vi "Car Wash.vi"() -> ()   [LabVIEW 2024]
doc: "Car wash\n\nWash entry : indicate empty or in use\nUser selects car wash options \nStart option\nCar wash indicator shows current step in car wash\nshows the elapsed time on indicator\nVehicle out of position indicator -> elapsed timer pause\n\nProgram start\nAll controls enabled\nWash entry green\n-> Wash vacant\nAll wash indicators turned off; elapsed time =0\nCar position slider Entry\n\nSelects wash options\nHigh pressure is the default\nStart -> starts the selected car wash options one by one\n\nShould disable all the wash options after start\nWash entry LED red -> Wash in Progress\n\nCheck if the car is in position\n\nUpon completing car wash step; if car is in position, go to next car wash step\n\nOnce all car wash steps are complete, vehicle out of position should turn green. User moves car position slider to exit car wash indicators off\nCar position slider -> Entry\nWash entry green and wash vacant\nWash entry cinsole options enabled"
uses:
  Controls/Wash Options.ctl
  Controls/Car Wash Indicators.ctl
  Controls/States.ctl
panel:
  out "Output":T2 {"Elapsed Time" format="%0.2f"}
  in  "Start":bool
  in  "stop":bool
  in  "Wash Options":T3
  in  "Car Position Slider":u8(slide) max=3 scale=0.0..4.0
  # "Entry Console"
  # "Car Wash Display"
  # "Car Position Simulation"
  # "Pre-Soak\nH-P Wash\nL-P Wax\nSpot Free Rinse"
  # "Underbody Wash\nBug Remover"
  # "Tire Shine\nAir Dry"
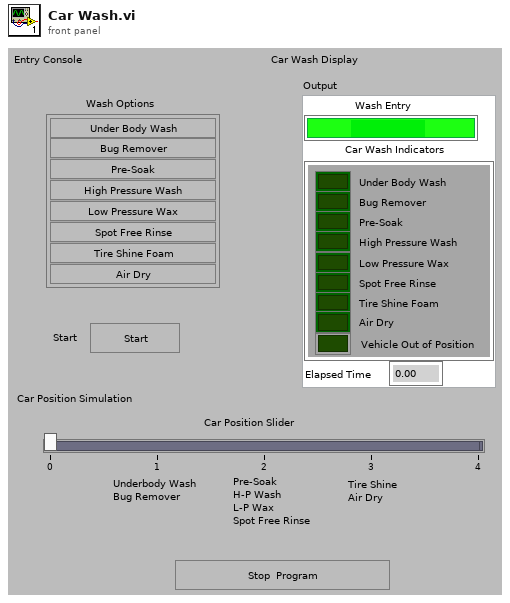
[diagram p1: front panel]
types:
  T1 = typedef "Car Wash Indicators.ctl" = cluster{"Under Body Wash":bool, "Bug Remover":bool, "Pre-Soak":bool, "High Pressure Wash":bool, "Low Pressure Wax":bool, "Spot Free Rinse":bool, "Tire Shine Foam":bool, "Air Dry":bool, "Vehicle Out of Position":bool}
  T2 = cluster{"Wash Entry":bool, "Car Wash Indicators":T1, "Elapsed Time":dbl}
  T3 = typedef "Wash Options.ctl" = cluster{"Underbody Wash":bool, "Bug Remover":bool, "Pre-Soak":bool, "High Pressure Wash":bool, "Low Pressure Wax":bool, "Spot Free Rinse":bool, "Tire Shine Foam":bool, "Air Dry":bool}
  T4 = cluster{"Start":refnum<vi>, "Wash Options":refnum<vi>, "Car Position Slider":refnum<vi>, "Wash Entry":refnum<vi>, "Elapsed Time":refnum<vi>}
  T5 = typedef "States.ctl" = enum16{"Initialize", "Wait for Event", "Under Body Wash", "Bug Remover", "Pre-Soak", "High Pressure Wash", "Low Pressure Wax", "Spot Free Rinse", "Tire Shine Foam", "Exit", "Air Dry", "Stop"}
  T6 = enum8{"Enabled", "Disabled", "Disabled and Grayed Out"}
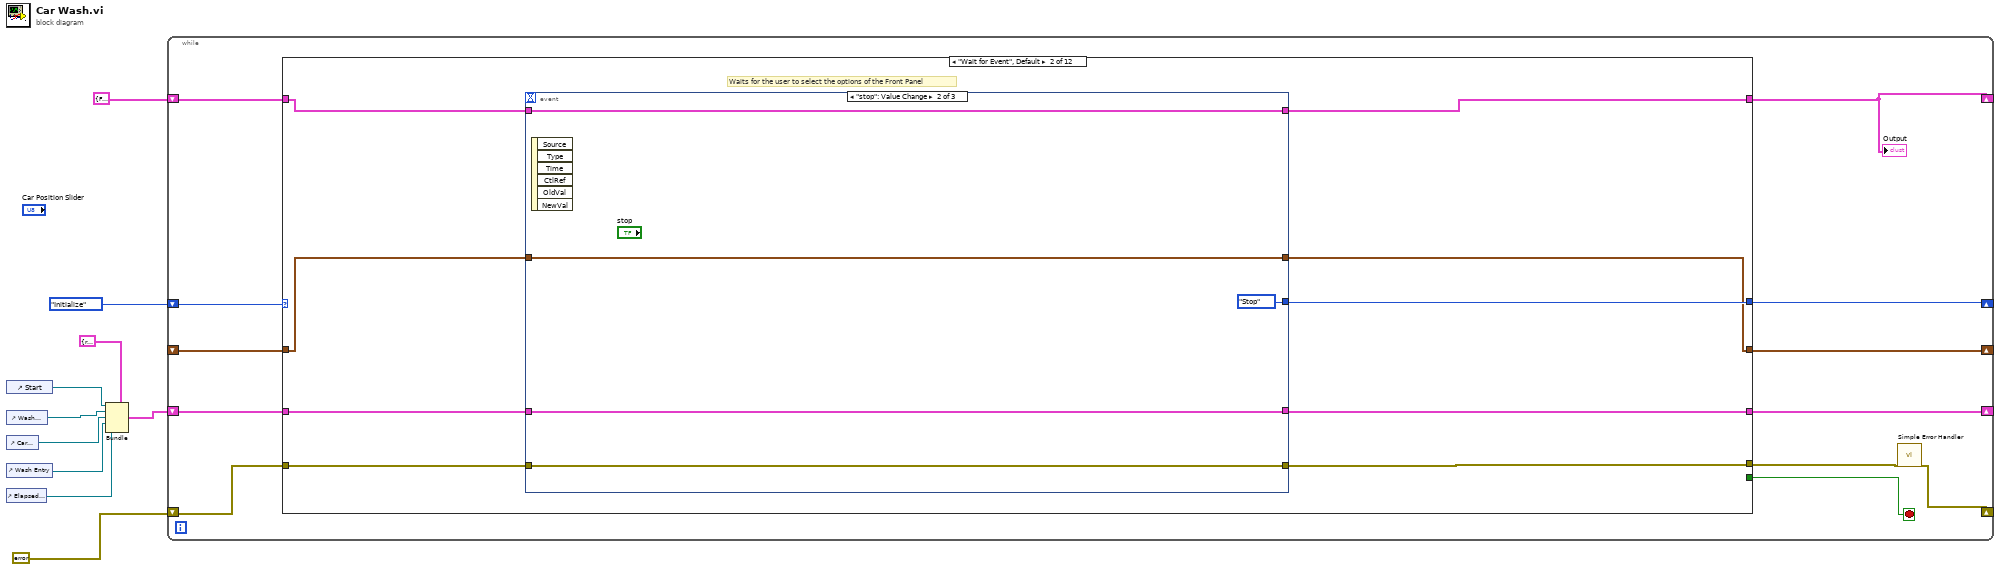
[diagram p0: block diagram]
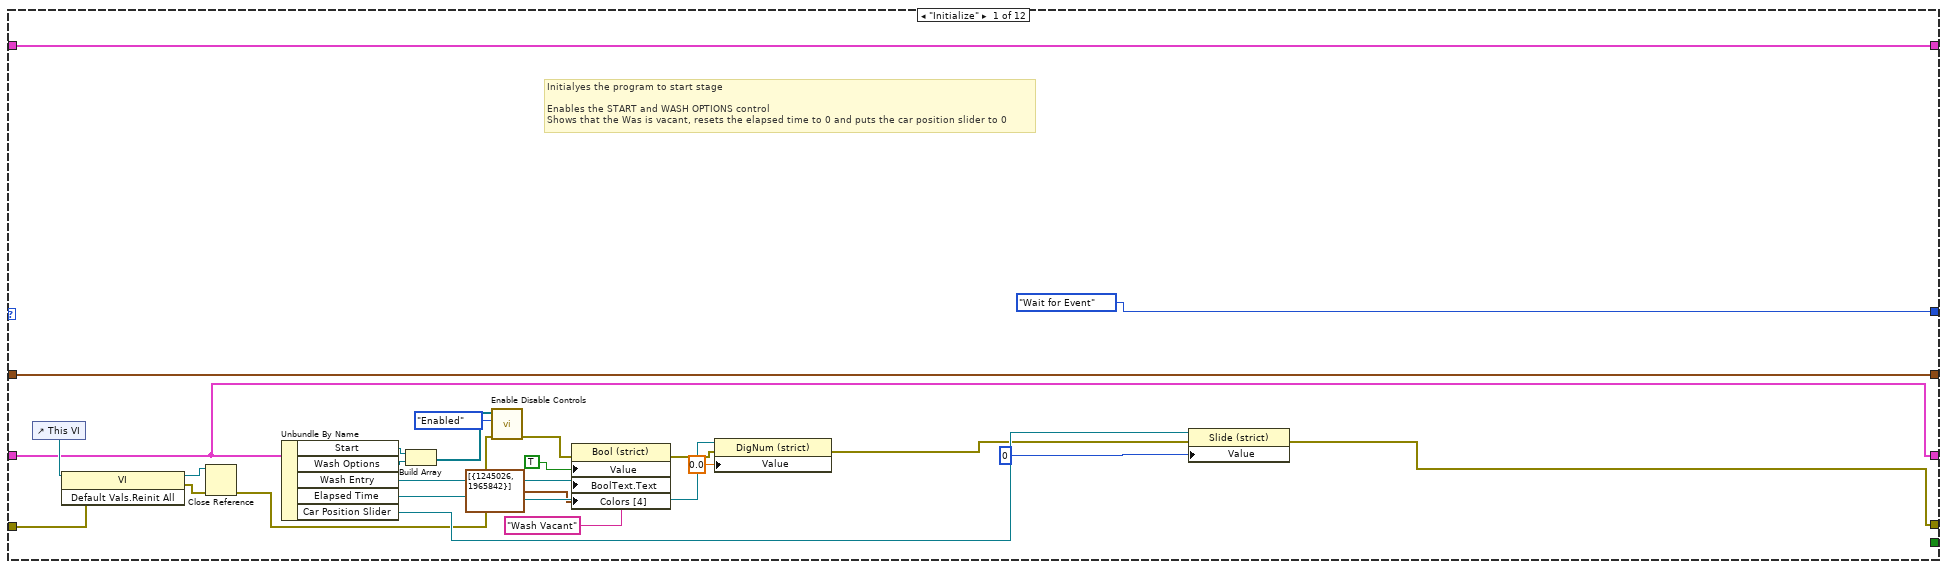
[diagram p2: hidden frame]
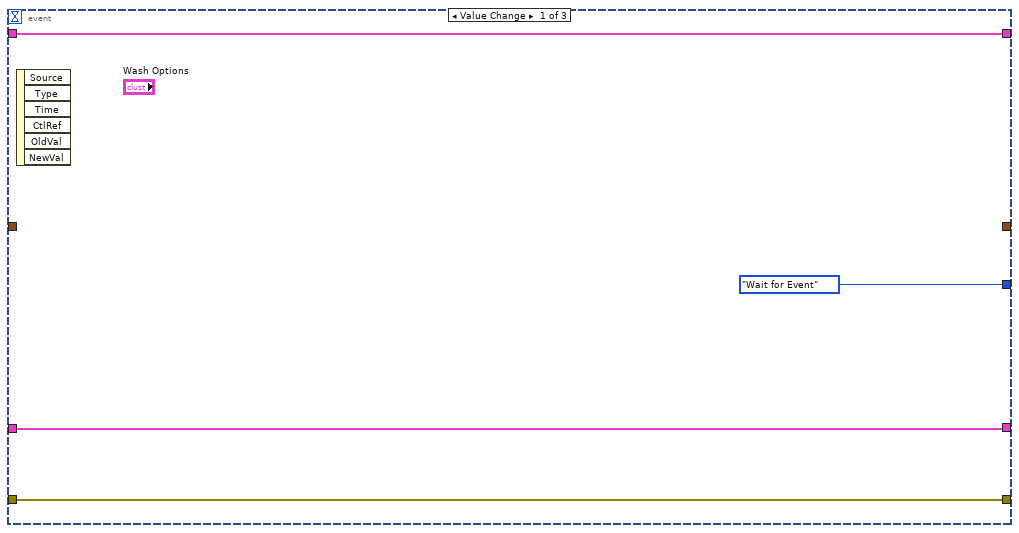
[diagram p3: hidden frame]
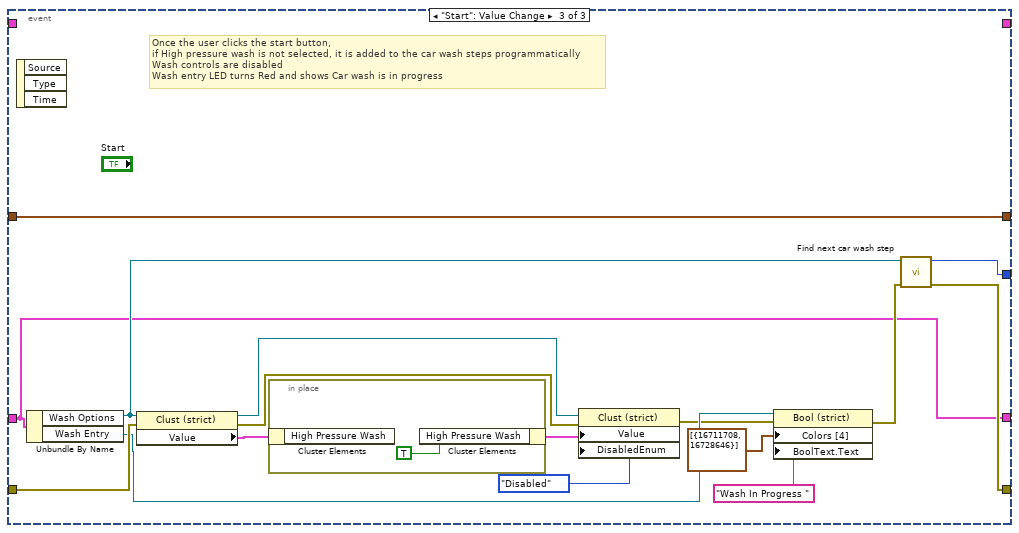
[diagram p4: hidden frame]
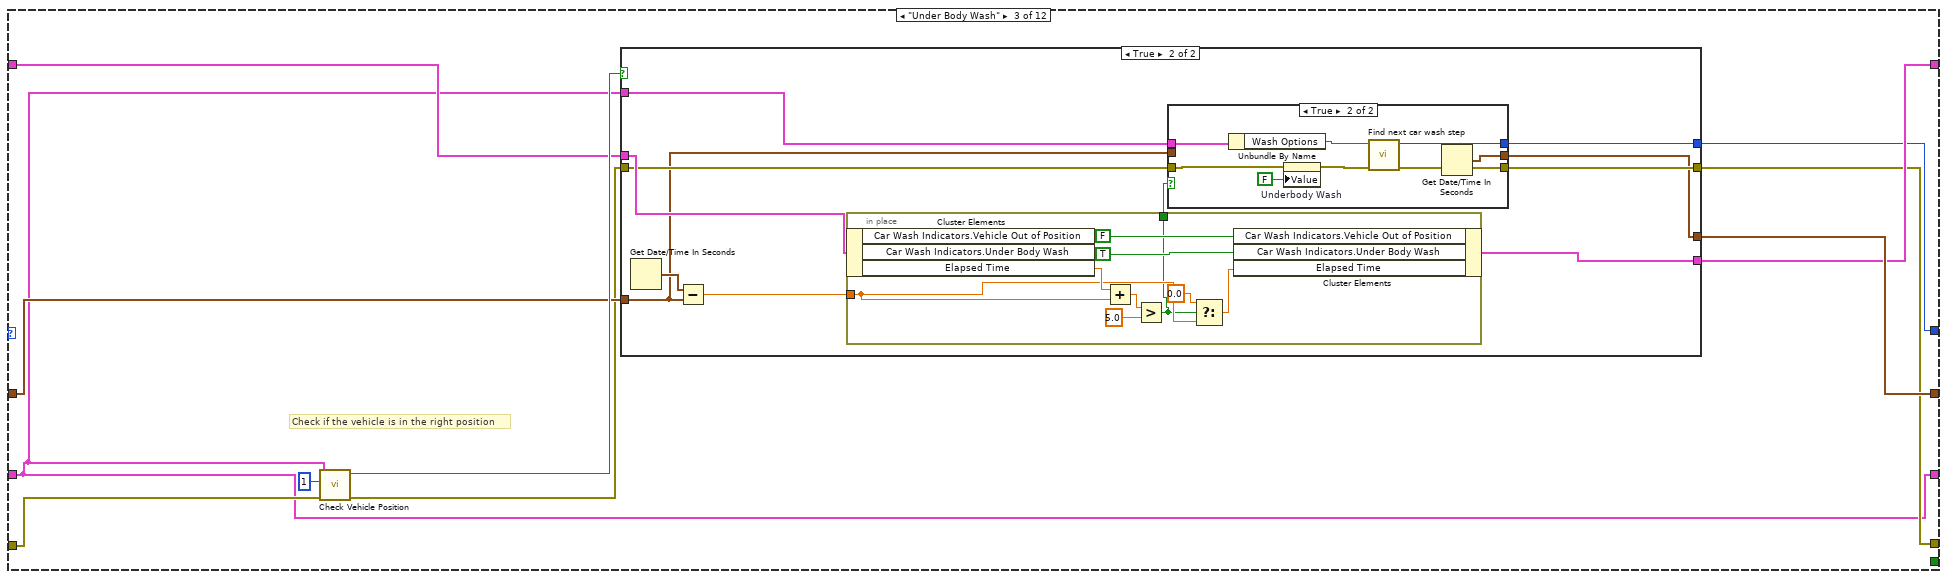
[diagram p5: hidden frame]
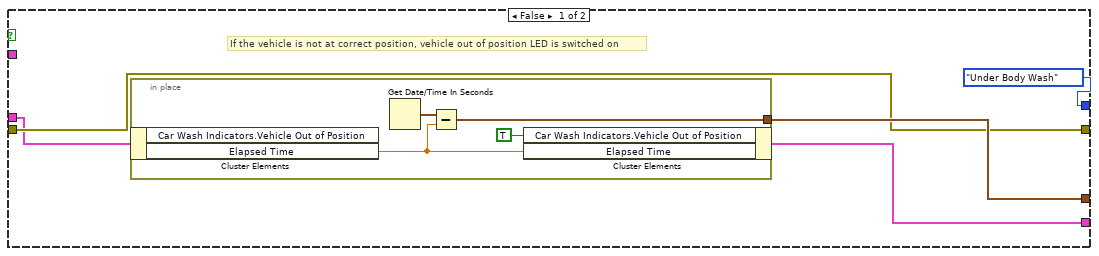
[diagram p6: hidden frame]
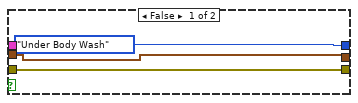
[diagram p7: hidden frame]
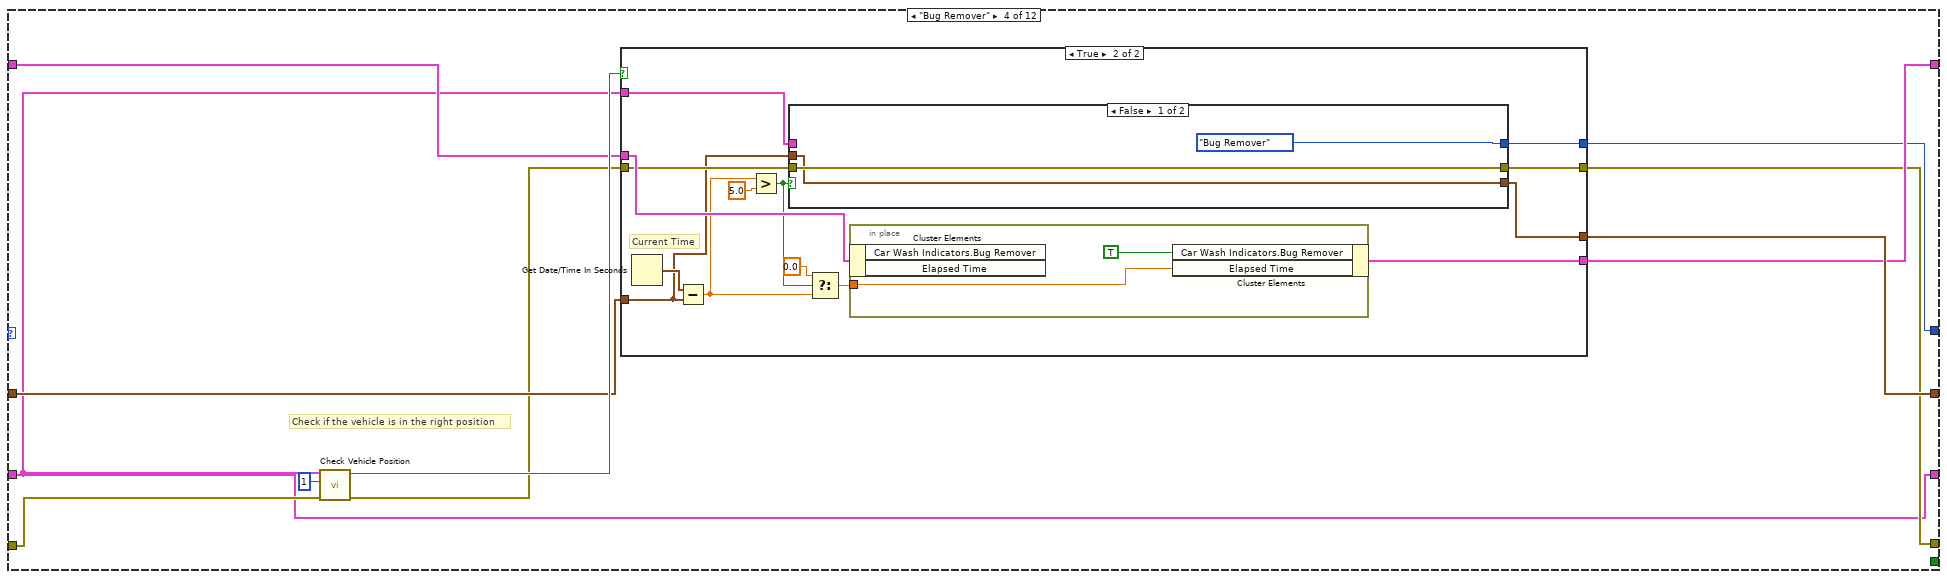
[diagram p8: hidden frame]
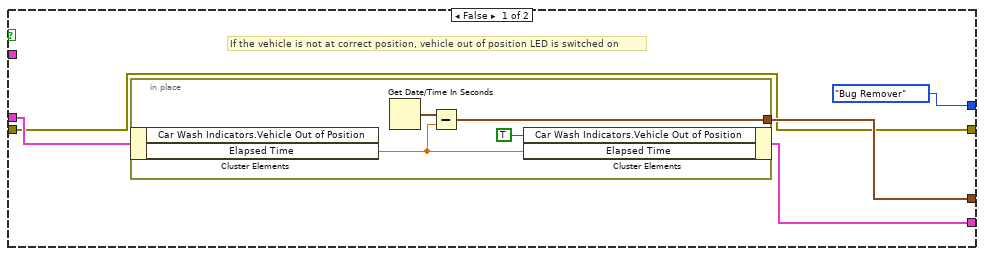
[diagram p9: hidden frame]
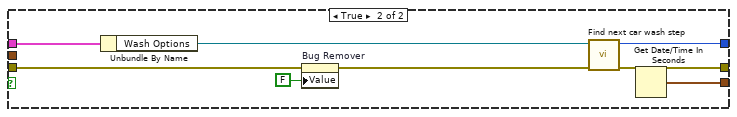
[diagram p10: hidden frame]
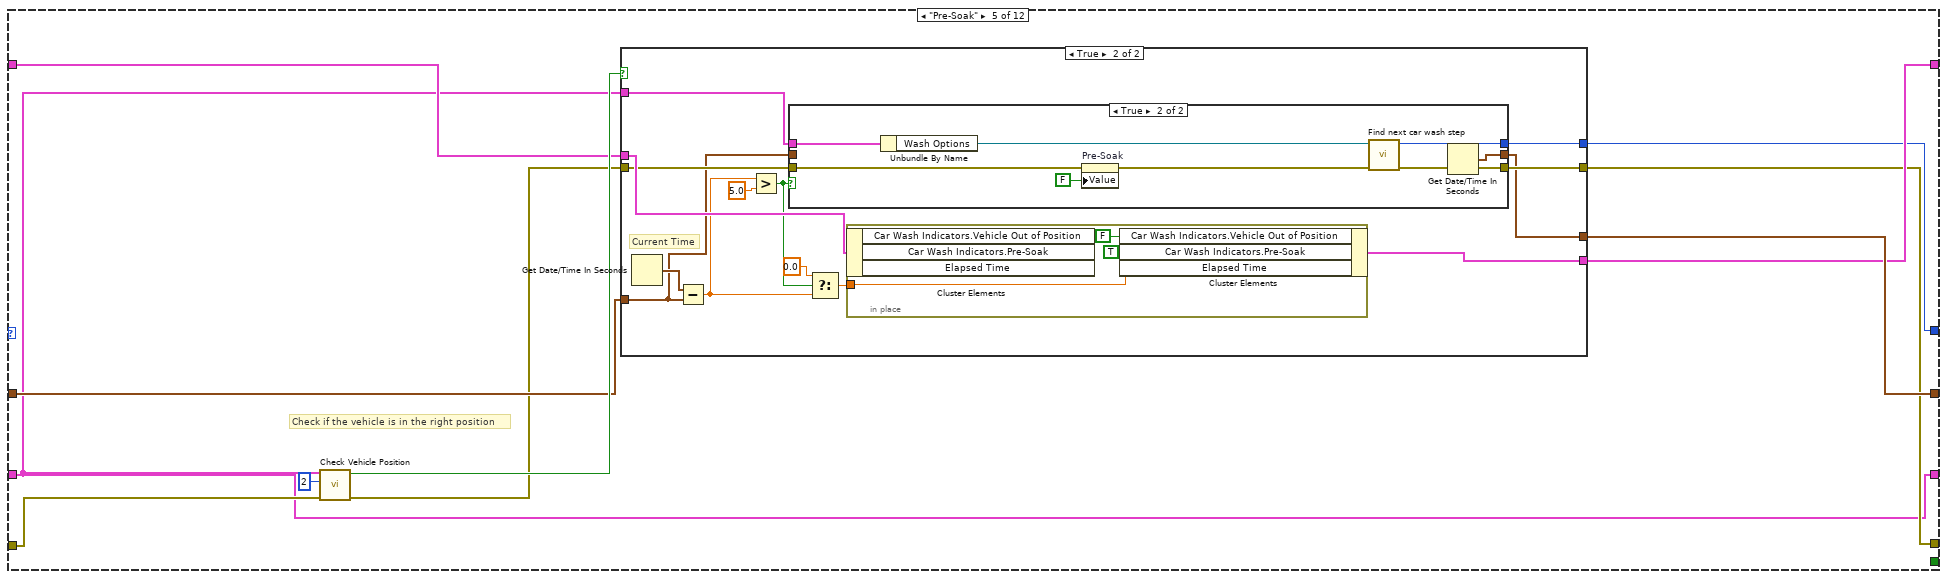
[diagram p11: hidden frame]
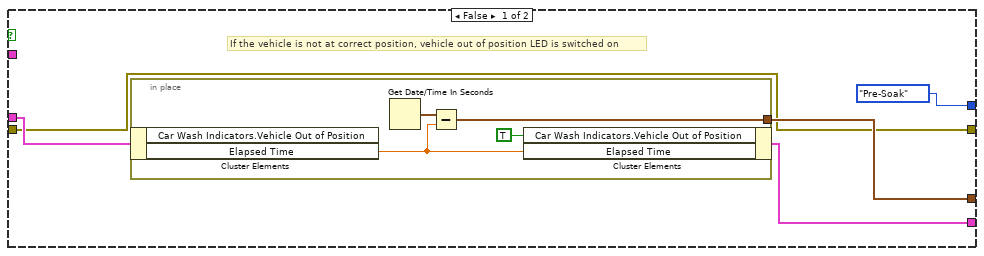
[diagram p12: hidden frame]
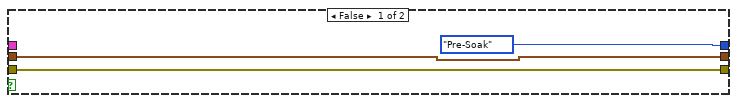
[diagram p13: hidden frame]
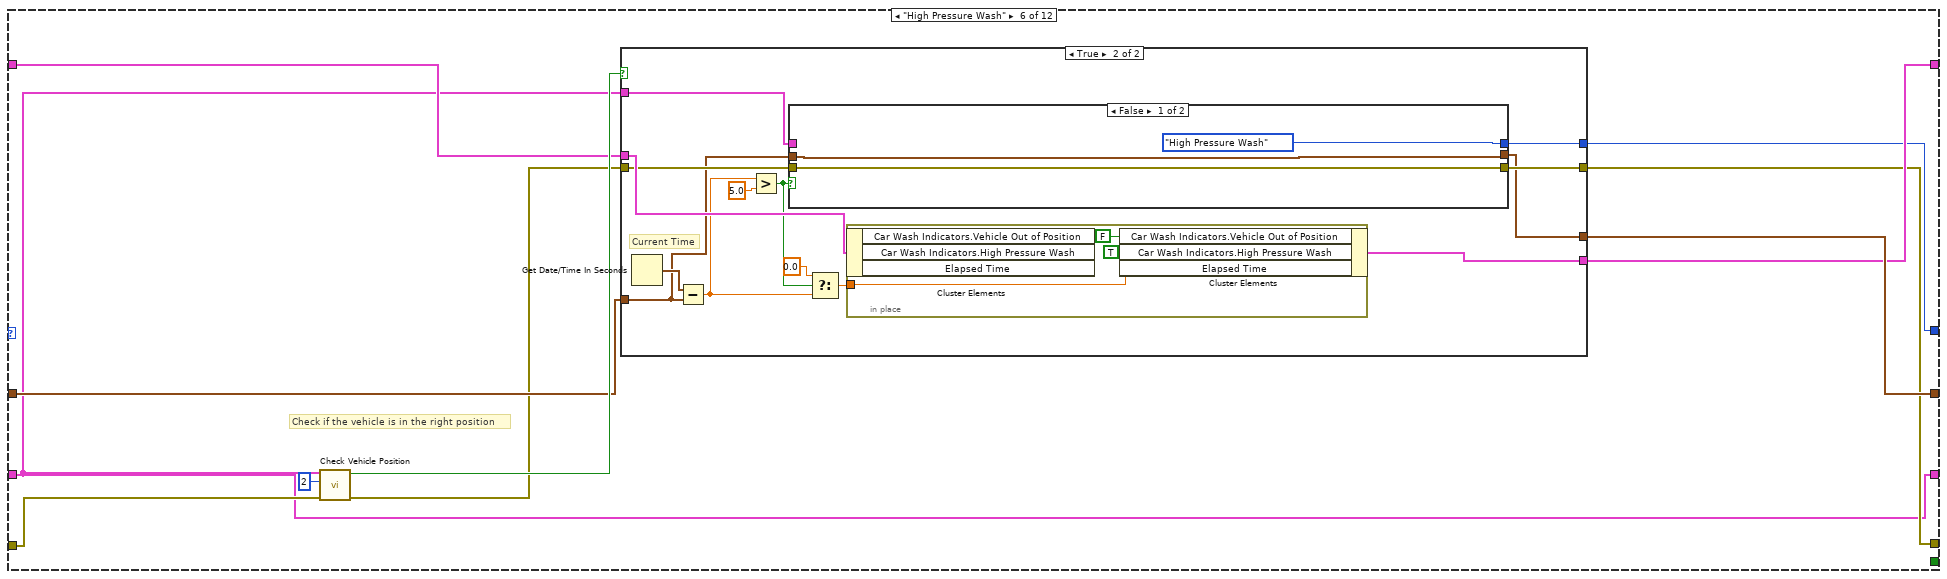
[diagram p14: hidden frame]
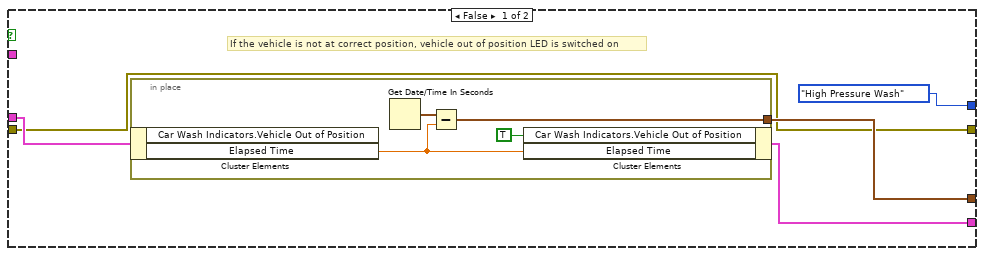
[diagram p15: hidden frame]
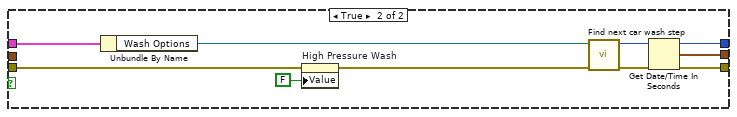
[diagram p16: hidden frame]
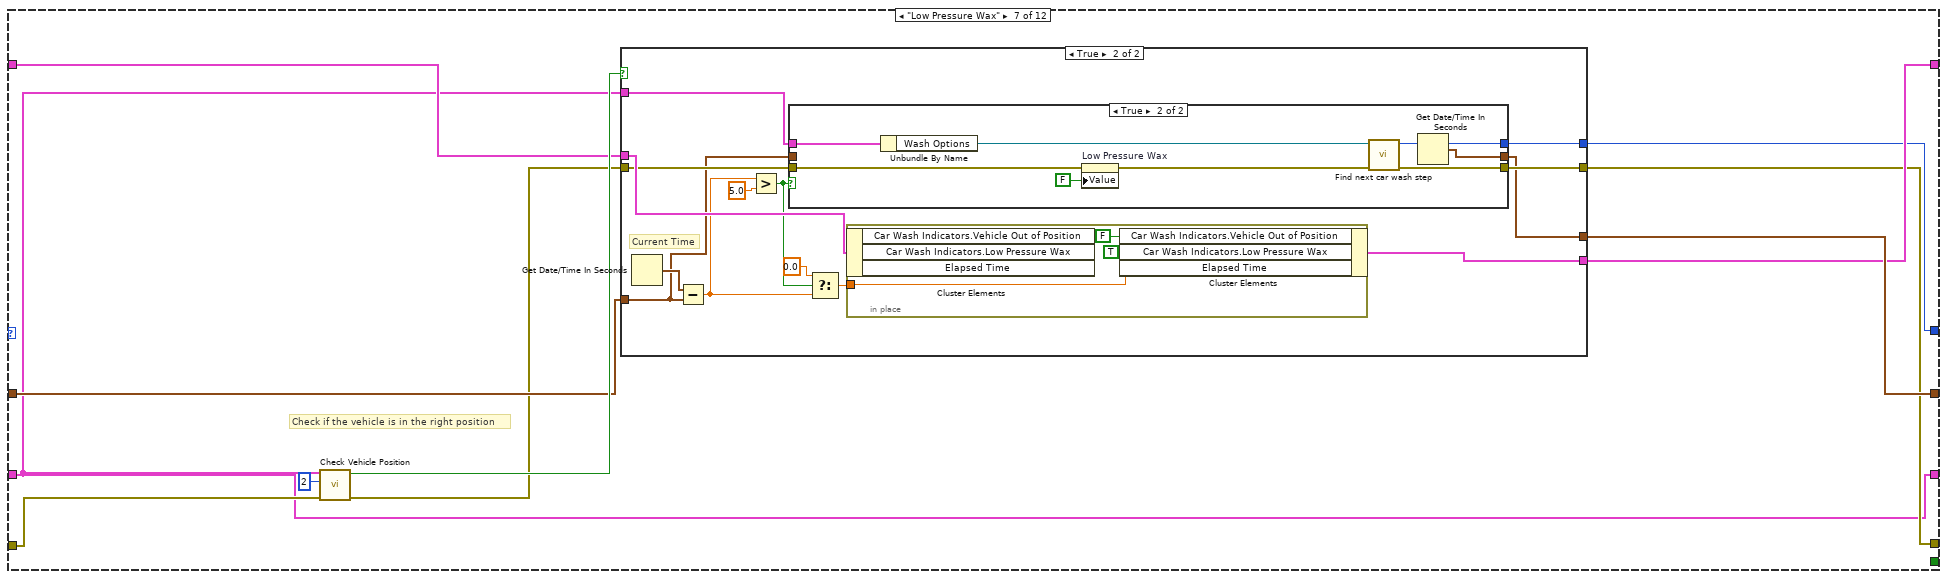
[diagram p17: hidden frame]
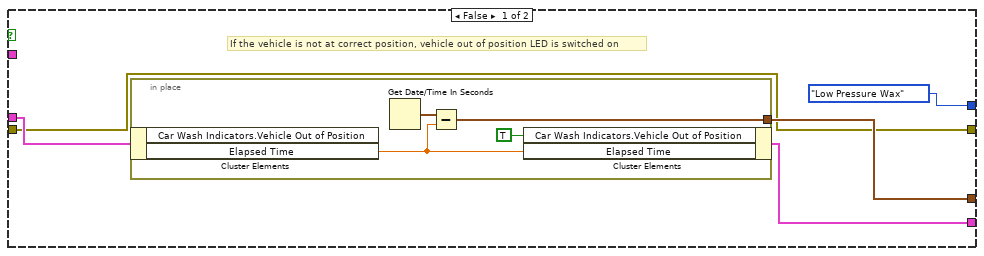
[diagram p18: hidden frame]
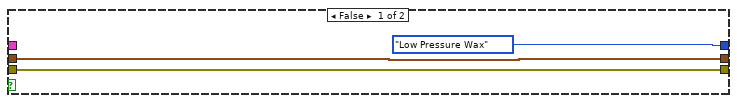
[diagram p19: hidden frame]
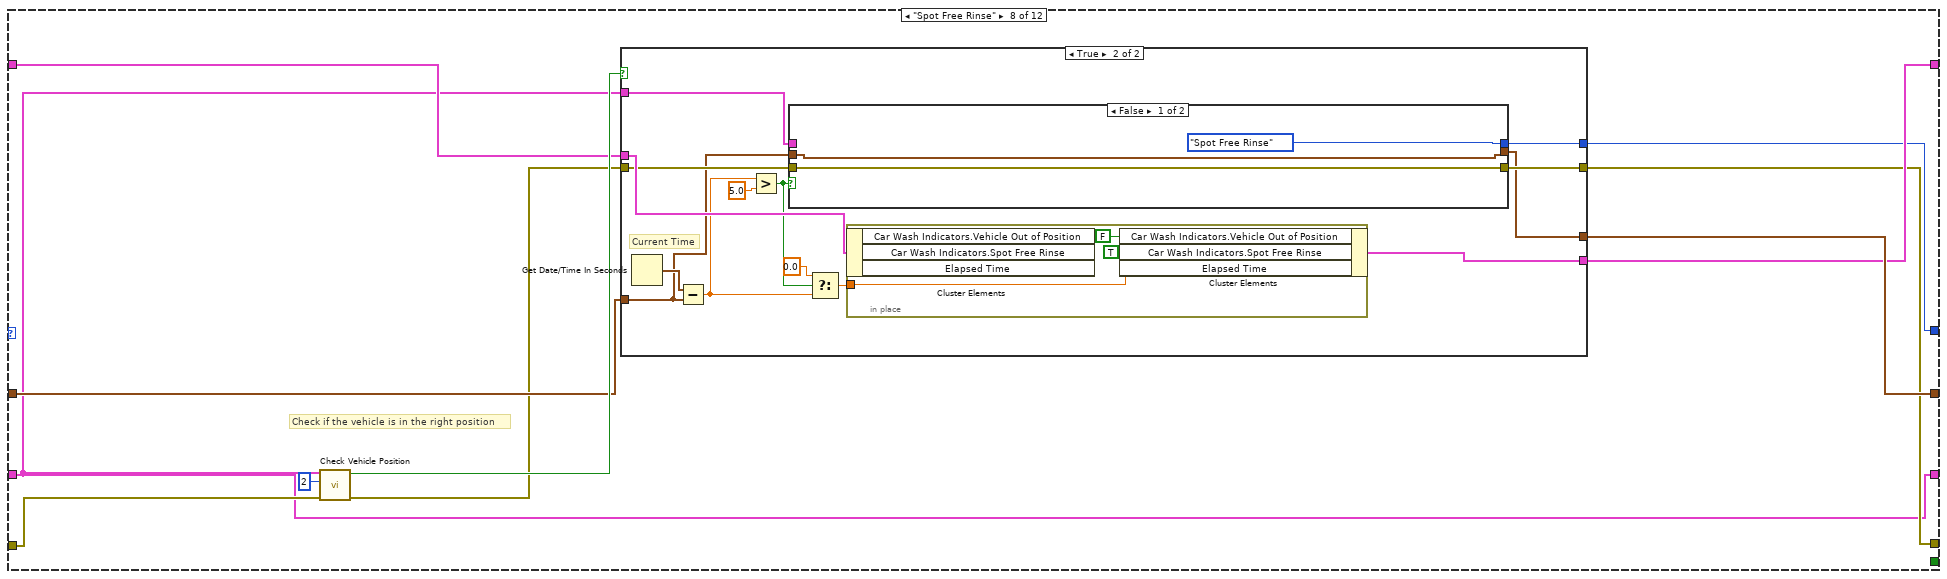
[diagram p20: hidden frame]
diagram:
  n1 = control-ref of="Start"() -> (w9:refnum<vi>)
  n2 = control-ref of="Wash Options"() -> (w8:refnum<vi>)
  n3 = control-ref of="Car Position Slider"() -> (w7:refnum<vi>)
  n4 = control-ref of="Wash Entry"() -> (w3:refnum<vi>)
  n5 = control-ref of="Elapsed Time"() -> (w2:refnum<vi>)
  n6 = Bundle(cluster=T4 {"Start"=refnum, "Wash Options"=refnum, "Car Position Slider"=refnum, "Wash Entry"=refnum, "Elapsed Time"=refnum}, "Start"=w9, "Wash Options"=w8, "Car Position Slider"=w7, "Wash Entry"=w3, "Elapsed Time"=w2) -> (w6:T4)
  n7 = while {
    shift-right: [w16] -> _
    shift-left: w6 -> [w21]
    shift-right: [w14] -> _
    shift-left: errorcluster {"status"=FALSE, "code"=0, "source"=""} ("error constant") -> [w20]
    shift-right: [w18] -> _
    shift-left: T2 {"Wash Entry"=FALSE, "Car Wash Indicators"={"Under Body Wash"=FALSE, "Bug Remover"=FALSE, "Pre-Soak"=FALSE, "High Pressure Wash"=FALSE, "Low Pressure Wax"=FALSE, "Spot Free Rinse"=FALSE, "Tire Shine Foam"=FALSE, "Air Dry"=FALSE, "Vehicle Out of Position"=FALSE}, "Elapsed Time"=0.0} ("Output") -> [w19]
    shift-right: [w17] -> _
    shift-left: States."Initialize" -> [w22]
    shift-right: [w12] -> _
    shift-left: _ -> [w13]
    stop <- w11 stop-if-true
    n8 = case shown="\"Wait for Event\", Default" w22 {
      tunnel: w21 -> [w23 w56 w83 w134 w181 w229 w277 w325 w373 w421 w471 w491]
      tunnel: w20 -> [w30 w55 w93 w144 w191 w239 w287 w335 w383 w431 w470 w501]
      tunnel: w19 -> [w33 w52 w91 w142 w189 w237 w285 w333 w381 w429 w476 w504]
      tunnel: [w34 w51 w84 w135 w182 w230 w278 w326 w374 w422 w477 w494] -> w15
      tunnel: [w33 w53 w88 w139 w186 w234 w282 w330 w378 w426 w476 w493] -> w18
      tunnel: [States."Wait for Event" w54 w87 w138 w185 w233 w281 w329 w377 w425 States."Wait for Event" w496] -> w17
      tunnel: [w23 w50 w83 w134 w181 w229 w277 w325 w373 w421 w471 w491] -> w16
      tunnel: w13 -> [w31 w49 w90 w141 w188 w236 w284 w332 w380 w428 w474 w492]
      tunnel: [w31 w48 w89 w140 w187 w235 w283 w331 w379 w427 w474 w492] -> w12
      tunnel: [_ _ _ _ _ _ _ _ _ _ TRUE ("stop 2") _] -> w11
      frame "Initialize" {
        # "Initialyes the program to start stage\n\nEnables the START and WASH OPTIONS control\nShows that the Was is vacant, resets the elapsed time to 0 and puts the car position slider to 0"
        n9 = control-ref of="This VI"() -> (w29:refnum<vi>)
        n10 = invoke class="VI" method="Default Vals.Reinit All"(reference=w29, error in=w30) -> (reference out=w24:refnum<vi>, error out=w26:errorcluster)  [unwired: 1 in, 1 out]
        n11 = Close Reference(reference=w24, error in (no error)=w26) -> (error out=w25:errorcluster)
        n12 = Unbundle By Name(w23) -> ("Start"=w47:refnum<vi>, "Wash Options"=w46:refnum<vi>, "Wash Entry"=w42:refnum<vi>, "Elapsed Time"=w40:refnum<vi>, "Car Position Slider"=w37:refnum<vi>)
        n13 = Build Array(w47, w46) -> (w45:refnum<vi>[])
        n14 = call "Enable Disable Controls.vi"("error in (no error)"=w25, "Disabled"=T6."Enabled", "Control Refnum"=w45) -> ("Error Out"=w43:errorcluster)  [unwired: 8 in]
        n15 = property class="Bool (strict)"(reference=w42, error in=w43, "Value"=TRUE, "BoolText.Text"="Wash Vacant" ("Boolean Text.Text"), "Colors [4]"=cluster{u32, u32}[] [{1245026, 1965842}]) -> (error out=w39:errorcluster)  [unwired: 1 out]
        n16 = property class="DigNum (strict)"(reference=w40, error in=w39, "Value"=0.0) -> (error out=w36:errorcluster)  [unwired: 1 out]
        n17 = property class="Slide (strict)"(reference=w37, error in=w36, "Value"=u8 0) -> (error out=w34:errorcluster)  [unwired: 1 out]
      }
      frame "Wait for Event", Default {
        # "Waits for the user to select the options of the Front Panel"
        n18 = event shown="[1] \"stop\": Value Change" {
          selector: _ -> [_ _ _]
          dyn-events: _ -> [_ _ _]
          timeout: _ -> [_ _ _]
          tunnel: w56 -> [w59 w62 w66]
          tunnel: w55 -> [w60 w63 w81]
          tunnel: [w60 w63 w70] -> w51
          tunnel: [w59 w62 w66] -> w50
          tunnel: [enum16{"Initialize", "Wait for Event"}."Wait for Event" States."Stop" ("Next Car Wash option") w69] -> w54
          tunnel: [w57 w64 _] -> w53
          tunnel: w52 -> [w57 w64 _]
          tunnel: w49 -> [_ w65 w67]
          tunnel: [_ w65 w67] -> w48
          event Value Change {
            n19 = event-data() -> ()  [unwired: 1 in, 6 out]
          }
          event "stop": Value Change {
            n20 = event-data() -> ()  [unwired: 1 in, 6 out]
          }
          event "Start": Value Change {
            # "Once the user clicks the start button,\nif High pressure wash is not selected, it is added to the car wash steps programmatically\nWash controls are disabled\nWash entry LED turns Red and shows Car wash is in progress"
            n21 = event-data() -> ()  [unwired: 1 in, 3 out]
            n22 = Unbundle By Name(w66) -> ("Wash Options"=w68:refnum<vi>, "Wash Entry"=w76:refnum<vi>)
            n23 = property class="Clust (strict)"(reference=w68, error in=w81) -> (reference out=w79:refnum<vi>, error out=w78:errorcluster, "Value"=w80:T3)
            n24 = in-place {
              n25 = in-place-cluster #1(w80) -> ()  [unwired: 1 out]
              n26 = in-place-cluster #1("High Pressure Wash"=TRUE) -> (w72:T3)
            }
            n27 = property class="Clust (strict)"(reference=w79, error in=w78, "Value"=w72, "DisabledEnum"=T6."Disabled" ("Disabled")) -> (error out=w75:errorcluster)  [unwired: 1 out]
            n28 = property class="Bool (strict)"(reference=w76, error in=w75, "Colors [4]"=cluster{u32, u32}[] [{16711708, 16728646}], "BoolText.Text"="Wash In Progress " ("Boolean Text.Text")) -> (error out=w71:errorcluster)  [unwired: 1 out]
            n29 = call "Find next car wash step.vi"("error in (no error)"=w71, "Control Refnum"=w68) -> ("error out"=w70:errorcluster, "Next Car Wash option"=w69:T5)  [unwired: 8 in]
          }
        }
      }
      frame "Under Body Wash" {
        # "Check if the vehicle is in the right position"
        n30 = call "Check Vehicle Position.vi"("error in (no error)"=w93, "Right Position"=u8 1, "Control Refnum"=w83) -> ("error out"=w85:errorcluster, "Vehicle in position"=w92:bool)  [unwired: 7 in]
        n31 = case shown="True" w92 {
          tunnel: w91 -> [w94 w113]
          tunnel: [w98 w112] -> w88
          tunnel: w90 -> [_ w103]
          tunnel: [w96 w106] -> w89
          tunnel: [States."Under Body Wash" w111] -> w87
          tunnel: w85 -> [w95 w110]
          tunnel: w83 -> [_ w108]
          tunnel: [w95 w109] -> w84
          frame False {
            # "If the vehicle is not at correct position, vehicle out of position LED is switched on"
            n32 = in-place {
              in-place-border: [w100] -> w96
              n33 = in-place-cluster #2(w94) -> ("Elapsed Time"=w99:dbl)  [unwired: 1 out]
              n34 = Get Date/Time In Seconds() -> (seconds since 1Jan1904=w101:timestamp)
              n35 = Subtract(x=w101, y=w99) -> (x-y=w100:timestamp)
              n36 = in-place-cluster #2("Car Wash Indicators.Vehicle Out of Position"=TRUE, "Elapsed Time"=w99) -> (w98:T2)
            }
          }
          frame True {
            n37 = Get Date/Time In Seconds() -> (seconds since 1Jan1904=w107:timestamp)
            n38 = Subtract(x=w107, y=w103) -> (x-y=w105:dbl)
            n39 = in-place {
              in-place-border: w105 -> [w129]
              in-place-border: [w125] -> w104
              n40 = in-place-cluster #3(w113) -> ("Elapsed Time"=w130:dbl)  [unwired: 2 out]
              n41 = Add(x=w130, y=w129) -> (x+y=w128:dbl)
              n42 = Greater?(x=w128, y=5.0) -> (0:w125:bool)
              n43 = Select(t=0.0, s=w125, f=w129) -> (s? t:f=w126:dbl)
              n44 = in-place-cluster #3("Car Wash Indicators.Vehicle Out of Position"=FALSE, "Car Wash Indicators.Under Body Wash"=TRUE, "Elapsed Time"=w126) -> (w112:T2)
            }
            n45 = case shown="True" w104 {
              tunnel: [States."Under Body Wash" w121] -> w111
              tunnel: w110 -> [w115 w123]
              tunnel: [w115 w120] -> w109
              tunnel: w108 -> [_ w119]
              tunnel: w103 -> [w114 _]
              tunnel: [w114 w117] -> w106
              frame False {
              }
              frame True {
                n46 = Unbundle By Name(w119) -> ("Wash Options"=w118:refnum<vi>)
                n47 = property on="Underbody Wash" class="Bool (strict)"(error in=w123, "Value"=FALSE) -> (error out=w122:errorcluster)  [unwired: 1 in, 1 out]
                n48 = call "Find next car wash step.vi"("error in (no error)"=w122, "Control Refnum"=w118) -> ("error out"=w120:errorcluster, "Next Car Wash option"=w121:T5)  [unwired: 8 in]
                n49 = Get Date/Time In Seconds() -> (seconds since 1Jan1904=w117:timestamp)
              }
            }
          }
        }
      }
      frame "Bug Remover" {
        # "Check if the vehicle is in the right position"
        n50 = call "Check Vehicle Position.vi"("error in (no error)"=w144, "Right Position"=u8 1, "Control Refnum"=w134) -> ("error out"=w136:errorcluster, "Vehicle in position"=w143:bool)  [unwired: 7 in]
        n51 = case shown="True" w143 {
          tunnel: w142 -> [w149 w167]
          tunnel: [w148 w166] -> w139
          tunnel: w141 -> [_ w155]
          tunnel: [w146 w154] -> w140
          tunnel: [States."Bug Remover" w160] -> w138
          tunnel: w136 -> [w145 w158]
          tunnel: w134 -> [_ w156]
          tunnel: [w145 w157] -> w135
          frame False {
            # "If the vehicle is not at correct position, vehicle out of position LED is switched on"
            n52 = in-place {
              in-place-border: [w151] -> w146
              n53 = in-place-cluster #4(w149) -> ("Elapsed Time"=w150:dbl)  [unwired: 1 out]
              n54 = Get Date/Time In Seconds() -> (seconds since 1Jan1904=w152:timestamp)
              n55 = Subtract(x=w152, y=w150) -> (x-y=w151:timestamp)
              n56 = in-place-cluster #4("Car Wash Indicators.Vehicle Out of Position"=TRUE, "Elapsed Time"=w150) -> (w148:T2)
            }
          }
          frame True {
            # "Current Time"
            n57 = Get Date/Time In Seconds() -> (seconds since 1Jan1904=w159:timestamp)
            n58 = Subtract(x=w159, y=w155) -> (x-y=w163:dbl)
            n59 = Greater?(x=w163, y=5.0) -> (0:w161:bool)
            n60 = case shown="False" w161 {
              tunnel: [States."Bug Remover" w175] -> w160
              tunnel: w158 -> [w169 w177]
              tunnel: [w169 w174] -> w157
              tunnel: w156 -> [_ w173]
              tunnel: w155 -> [w168 _]
              tunnel: [w168 w171] -> w154
              frame False {
              }
              frame True {
                n61 = Unbundle By Name(w173) -> ("Wash Options"=w172:refnum<vi>)
                n62 = property on="Bug Remover" class="Bool (strict)"(error in=w177, "Value"=FALSE) -> (error out=w176:errorcluster)  [unwired: 1 in, 1 out]
                n63 = call "Find next car wash step.vi"("error in (no error)"=w176, "Control Refnum"=w172) -> ("error out"=w174:errorcluster, "Next Car Wash option"=w175:T5)  [unwired: 8 in]
                n64 = Get Date/Time In Seconds() -> (seconds since 1Jan1904=w171:timestamp)
              }
            }
            n65 = Select(t=0.0, s=w161, f=w163) -> (s? t:f=w162:dbl)
            n66 = in-place {
              in-place-border: w162 -> [w179]
              n67 = in-place-cluster #5(w167) -> ()  [unwired: 2 out]
              n68 = in-place-cluster #5("Car Wash Indicators.Bug Remover"=TRUE ("Car Wash Indicators.Under Body Wash"), "Elapsed Time"=w179) -> (w166:T2)
            }
          }
        }
      }
      frame "Pre-Soak" {
        # "Check if the vehicle is in the right position"
        n69 = call "Check Vehicle Position.vi"("error in (no error)"=w191, "Right Position"=u8 2, "Control Refnum"=w181) -> ("error out"=w183:errorcluster, "Vehicle in position"=w190:bool)  [unwired: 7 in]
        n70 = case shown="True" w190 {
          tunnel: w189 -> [w196 w214]
          tunnel: [w195 w213] -> w186
          tunnel: w188 -> [_ w202]
          tunnel: [w193 w201] -> w187
          tunnel: [States."Pre-Soak" w207] -> w185
          tunnel: w183 -> [w192 w205]
          tunnel: w181 -> [_ w203]
          tunnel: [w192 w204] -> w182
          frame False {
            # "If the vehicle is not at correct position, vehicle out of position LED is switched on"
            n71 = in-place {
              in-place-border: [w198] -> w193
              n72 = in-place-cluster #6(w196) -> ("Elapsed Time"=w197:dbl)  [unwired: 1 out]
              n73 = Get Date/Time In Seconds() -> (seconds since 1Jan1904=w199:timestamp)
              n74 = Subtract(x=w199, y=w197) -> (x-y=w198:timestamp)
              n75 = in-place-cluster #6("Car Wash Indicators.Vehicle Out of Position"=TRUE, "Elapsed Time"=w197) -> (w195:T2)
            }
          }
          frame True {
            # "Current Time"
            n76 = Get Date/Time In Seconds() -> (seconds since 1Jan1904=w206:timestamp)
            n77 = Subtract(x=w206, y=w202) -> (x-y=w210:dbl)
            n78 = Greater?(x=w210, y=5.0) -> (0:w208:bool)
            n79 = case shown="True" w208 {
              tunnel: [States."Pre-Soak" w222] -> w207
              tunnel: w205 -> [w216 w224]
              tunnel: [w216 w221] -> w204
              tunnel: w203 -> [_ w220]
              tunnel: w202 -> [w215 _]
              tunnel: [w215 w218] -> w201
              frame False {
              }
              frame True {
                n80 = Unbundle By Name(w220) -> ("Wash Options"=w219:refnum<vi>)
                n81 = property on="Pre-Soak" class="Bool (strict)"(error in=w224, "Value"=FALSE) -> (error out=w223:errorcluster)  [unwired: 1 in, 1 out]
                n82 = call "Find next car wash step.vi"("error in (no error)"=w223, "Control Refnum"=w219) -> ("error out"=w221:errorcluster, "Next Car Wash option"=w222:T5)  [unwired: 8 in]
                n83 = Get Date/Time In Seconds() -> (seconds since 1Jan1904=w218:timestamp)
              }
            }
            n84 = Select(t=0.0, s=w208, f=w210) -> (s? t:f=w209:dbl)
            n85 = in-place {
              in-place-border: w209 -> [w227]
              n86 = in-place-cluster #7(w214) -> ()  [unwired: 3 out]
              n87 = in-place-cluster #7("Car Wash Indicators.Vehicle Out of Position"=FALSE, "Car Wash Indicators.Pre-Soak"=TRUE ("Car Wash Indicators.Under Body Wash"), "Elapsed Time"=w227) -> (w213:T2)
            }
          }
        }
      }
      frame "High Pressure Wash" {
        # "Check if the vehicle is in the right position"
        n88 = call "Check Vehicle Position.vi"("error in (no error)"=w239, "Right Position"=u8 2, "Control Refnum"=w229) -> ("error out"=w231:errorcluster, "Vehicle in position"=w238:bool)  [unwired: 7 in]
        n89 = case shown="True" w238 {
          tunnel: w237 -> [w244 w262]
          tunnel: [w243 w261] -> w234
          tunnel: w236 -> [_ w250]
          tunnel: [w241 w249] -> w235
          tunnel: [States."High Pressure Wash" w255] -> w233
          tunnel: w231 -> [w240 w253]
          tunnel: w229 -> [_ w251]
          tunnel: [w240 w252] -> w230
          frame False {
            # "If the vehicle is not at correct position, vehicle out of position LED is switched on"
            n90 = in-place {
              in-place-border: [w246] -> w241
              n91 = in-place-cluster #8(w244) -> ("Elapsed Time"=w245:dbl)  [unwired: 1 out]
              n92 = Get Date/Time In Seconds() -> (seconds since 1Jan1904=w247:timestamp)
              n93 = Subtract(x=w247, y=w245) -> (x-y=w246:timestamp)
              n94 = in-place-cluster #8("Car Wash Indicators.Vehicle Out of Position"=TRUE, "Elapsed Time"=w245) -> (w243:T2)
            }
          }
          frame True {
            # "Current Time"
            n95 = Get Date/Time In Seconds() -> (seconds since 1Jan1904=w254:timestamp)
            n96 = Subtract(x=w254, y=w250) -> (x-y=w258:dbl)
            n97 = Greater?(x=w258, y=5.0) -> (0:w256:bool)
            n98 = case shown="False" w256 {
              tunnel: [States."High Pressure Wash" w270] -> w255
              tunnel: w253 -> [w264 w272]
              tunnel: [w264 w269] -> w252
              tunnel: w251 -> [_ w268]
              tunnel: w250 -> [w263 _]
              tunnel: [w263 w266] -> w249
              frame False {
              }
              frame True {
                n99 = Unbundle By Name(w268) -> ("Wash Options"=w267:refnum<vi>)
                n100 = property on="High Pressure Wash" class="Bool (strict)"(error in=w272, "Value"=FALSE) -> (error out=w271:errorcluster)  [unwired: 1 in, 1 out]
                n101 = call "Find next car wash step.vi"("error in (no error)"=w271, "Control Refnum"=w267) -> ("error out"=w269:errorcluster, "Next Car Wash option"=w270:T5)  [unwired: 8 in]
                n102 = Get Date/Time In Seconds() -> (seconds since 1Jan1904=w266:timestamp)
              }
            }
            n103 = Select(t=0.0, s=w256, f=w258) -> (s? t:f=w257:dbl)
            n104 = in-place {
              in-place-border: w257 -> [w275]
              n105 = in-place-cluster #9(w262) -> ()  [unwired: 3 out]
              n106 = in-place-cluster #9("Car Wash Indicators.Vehicle Out of Position"=FALSE, "Car Wash Indicators.High Pressure Wash"=TRUE ("Car Wash Indicators.Under Body Wash"), "Elapsed Time"=w275) -> (w261:T2)
            }
          }
        }
      }
      frame "Low Pressure Wax" {
        # "Check if the vehicle is in the right position"
        n107 = call "Check Vehicle Position.vi"("error in (no error)"=w287, "Right Position"=u8 2, "Control Refnum"=w277) -> ("error out"=w279:errorcluster, "Vehicle in position"=w286:bool)  [unwired: 7 in]
        n108 = case shown="True" w286 {
          tunnel: w285 -> [w292 w310]
          tunnel: [w291 w309] -> w282
          tunnel: w284 -> [_ w298]
          tunnel: [w289 w297] -> w283
          tunnel: [States."Low Pressure Wax" w303] -> w281
          tunnel: w279 -> [w288 w301]
          tunnel: w277 -> [_ w299]
          tunnel: [w288 w300] -> w278
          frame False {
            # "If the vehicle is not at correct position, vehicle out of position LED is switched on"
            n109 = in-place {
              in-place-border: [w294] -> w289
              n110 = in-place-cluster #10(w292) -> ("Elapsed Time"=w293:dbl)  [unwired: 1 out]
              n111 = Get Date/Time In Seconds() -> (seconds since 1Jan1904=w295:timestamp)
              n112 = Subtract(x=w295, y=w293) -> (x-y=w294:timestamp)
              n113 = in-place-cluster #10("Car Wash Indicators.Vehicle Out of Position"=TRUE, "Elapsed Time"=w293) -> (w291:T2)
            }
          }
          frame True {
            # "Current Time"
            n114 = Get Date/Time In Seconds() -> (seconds since 1Jan1904=w302:timestamp)
            n115 = Subtract(x=w302, y=w298) -> (x-y=w306:dbl)
            n116 = Greater?(x=w306, y=5.0) -> (0:w304:bool)
            n117 = case shown="True" w304 {
              tunnel: [States."Low Pressure Wax" w318] -> w303
              tunnel: w301 -> [w312 w320]
              tunnel: [w312 w317] -> w300
              tunnel: w299 -> [_ w316]
              tunnel: w298 -> [w311 _]
              tunnel: [w311 w314] -> w297
              frame False {
              }
              frame True {
                n118 = Unbundle By Name(w316) -> ("Wash Options"=w315:refnum<vi>)
                n119 = property on="Low Pressure Wax" class="Bool (strict)"(error in=w320, "Value"=FALSE) -> (error out=w319:errorcluster)  [unwired: 1 in, 1 out]
                n120 = call "Find next car wash step.vi"("error in (no error)"=w319, "Control Refnum"=w315) -> ("error out"=w317:errorcluster, "Next Car Wash option"=w318:T5)  [unwired: 8 in]
                n121 = Get Date/Time In Seconds() -> (seconds since 1Jan1904=w314:timestamp)
              }
            }
            n122 = Select(t=0.0, s=w304, f=w306) -> (s? t:f=w305:dbl)
            n123 = in-place {
              in-place-border: w305 -> [w323]
              n124 = in-place-cluster #11(w310) -> ()  [unwired: 3 out]
              n125 = in-place-cluster #11("Car Wash Indicators.Vehicle Out of Position"=FALSE, "Car Wash Indicators.Low Pressure Wax"=TRUE ("Car Wash Indicators.Under Body Wash"), "Elapsed Time"=w323) -> (w309:T2)
            }
          }
        }
      }
      frame "Spot Free Rinse" {
        # "Check if the vehicle is in the right position"
        n126 = call "Check Vehicle Position.vi"("error in (no error)"=w335, "Right Position"=u8 2, "Control Refnum"=w325) -> ("error out"=w327:errorcluster, "Vehicle in position"=w334:bool)  [unwired: 7 in]
        n127 = case shown="True" w334 {
          tunnel: w333 -> [w340 w358]
          tunnel: [w339 w357] -> w330
          tunnel: w332 -> [_ w346]
          tunnel: [w337 w345] -> w331
          tunnel: [States."Spot Free Rinse" w351] -> w329
          tunnel: w327 -> [w336 w349]
          tunnel: w325 -> [_ w347]
          tunnel: [w336 w348] -> w326
          frame False {
            # "If the vehicle is not at correct position, vehicle out of position LED is switched on"
            n128 = in-place {
              in-place-border: [w342] -> w337
              n129 = in-place-cluster #12(w340) -> ("Elapsed Time"=w341:dbl)  [unwired: 1 out]
              n130 = Get Date/Time In Seconds() -> (seconds since 1Jan1904=w343:timestamp)
              n131 = Subtract(x=w343, y=w341) -> (x-y=w342:timestamp)
              n132 = in-place-cluster #12("Car Wash Indicators.Vehicle Out of Position"=TRUE, "Elapsed Time"=w341) -> (w339:T2)
            }
          }
          frame True {
            # "Current Time"
            n133 = Get Date/Time In Seconds() -> (seconds since 1Jan1904=w350:timestamp)
            n134 = Subtract(x=w350, y=w346) -> (x-y=w354:dbl)
            n135 = Greater?(x=w354, y=5.0) -> (0:w352:bool)
            n136 = case shown="False" w352 {
              tunnel: [States."Spot Free Rinse" w366] -> w351
              tunnel: w349 -> [w360 w368]
              tunnel: [w360 w365] -> w348
              tunnel: w347 -> [_ w364]
              tunnel: [w359 w362] -> w345
              tunnel: w346 -> [w359 _]
              frame False {
              }
              frame True {
                n137 = Unbundle By Name(w364) -> ("Wash Options"=w363:refnum<vi>)
                n138 = property on="Spot Free Rinse" class="Bool (strict)"(error in=w368, "Value"=FALSE) -> (error out=w367:errorcluster)  [unwired: 1 in, 1 out]
                n139 = call "Find next car wash step.vi"("error in (no error)"=w367, "Control Refnum"=w363) -> ("error out"=w365:errorcluster, "Next Car Wash option"=w366:T5)  [unwired: 8 in]
                n140 = Get Date/Time In Seconds() -> (seconds since 1Jan1904=w362:timestamp)
              }
            }
            n141 = Select(t=0.0, s=w352, f=w354) -> (s? t:f=w353:dbl)
            n142 = in-place {
              in-place-border: w353 -> [w371]
              n143 = in-place-cluster #13(w358) -> ()  [unwired: 3 out]
              n144 = in-place-cluster #13("Car Wash Indicators.Vehicle Out of Position"=FALSE, "Car Wash Indicators.Spot Free Rinse"=TRUE ("Car Wash Indicators.Under Body Wash"), "Elapsed Time"=w371) -> (w357:T2)
            }
          }
        }
      }
      frame "Tire Shine Foam" {
        # "Check if the vehicle is in the right position"
        n145 = call "Check Vehicle Position.vi"("error in (no error)"=w383, "Right Position"=u8 3, "Control Refnum"=w373) -> ("error out"=w375:errorcluster, "Vehicle in position"=w382:bool)  [unwired: 7 in]
        n146 = case shown="True" w382 {
          tunnel: w381 -> [w388 w406]
          tunnel: [w387 w405] -> w378
          tunnel: w380 -> [_ w394]
          tunnel: [w385 w393] -> w379
          tunnel: [States."Tire Shine Foam" w399] -> w377
          tunnel: w375 -> [w384 w397]
          tunnel: w373 -> [_ w395]
          tunnel: [w384 w396] -> w374
          frame False {
            # "If the vehicle is not at correct position, vehicle out of position LED is switched on"
            n147 = in-place {
              in-place-border: [w390] -> w385
              n148 = in-place-cluster #14(w388) -> ("Elapsed Time"=w389:dbl)  [unwired: 1 out]
              n149 = Get Date/Time In Seconds() -> (seconds since 1Jan1904=w391:timestamp)
              n150 = Subtract(x=w391, y=w389) -> (x-y=w390:timestamp)
              n151 = in-place-cluster #14("Car Wash Indicators.Vehicle Out of Position"=TRUE, "Elapsed Time"=w389) -> (w387:T2)
            }
          }
          frame True {
            # "Current Time"
            n152 = Get Date/Time In Seconds() -> (seconds since 1Jan1904=w398:timestamp)
            n153 = Subtract(x=w398, y=w394) -> (x-y=w402:dbl)
            n154 = Greater?(x=w402, y=5.0) -> (0:w400:bool)
            n155 = case shown="True" w400 {
              tunnel: [States."Tire Shine Foam" w414] -> w399
              tunnel: w397 -> [w408 w416]
              tunnel: [w408 w413] -> w396
              tunnel: w395 -> [_ w412]
              tunnel: w394 -> [w407 _]
              tunnel: [w407 w410] -> w393
              frame False {
              }
              frame True {
                n156 = Unbundle By Name(w412) -> ("Wash Options"=w411:refnum<vi>)
                n157 = property on="Tire Shine Foam" class="Bool (strict)"(error in=w416, "Value"=FALSE) -> (error out=w415:errorcluster)  [unwired: 1 in, 1 out]
                n158 = call "Find next car wash step.vi"("error in (no error)"=w415, "Control Refnum"=w411) -> ("error out"=w413:errorcluster, "Next Car Wash option"=w414:T5)  [unwired: 8 in]
                n159 = Get Date/Time In Seconds() -> (seconds since 1Jan1904=w410:timestamp)
              }
            }
            n160 = Select(t=0.0, s=w400, f=w402) -> (s? t:f=w401:dbl)
            n161 = in-place {
              in-place-border: w401 -> [w419]
              n162 = in-place-cluster #15(w406) -> ()  [unwired: 3 out]
              n163 = in-place-cluster #15("Car Wash Indicators.Vehicle Out of Position"=FALSE, "Car Wash Indicators.Tire Shine Foam"=TRUE ("Car Wash Indicators.Under Body Wash"), "Elapsed Time"=w419) -> (w405:T2)
            }
          }
        }
      }
      frame "Air Dry" {
        # "Check if the vehicle is in the right position"
        n164 = call "Check Vehicle Position.vi"("error in (no error)"=w431, "Right Position"=u8 3, "Control Refnum"=w421) -> ("error out"=w423:errorcluster, "Vehicle in position"=w430:bool)  [unwired: 7 in]
        n165 = case shown="True" w430 {
          tunnel: w429 -> [w436 w454]
          tunnel: [w435 w453] -> w426
          tunnel: w428 -> [_ w441]
          tunnel: [w433 w442] -> w427
          tunnel: [States."Air Dry" w447] -> w425
          tunnel: w423 -> [w432 w445]
          tunnel: w421 -> [_ w443]
          tunnel: [w432 w444] -> w422
          frame False {
            # "If the vehicle is not at correct position, vehicle out of position LED is switched on"
            n166 = in-place {
              in-place-border: [w438] -> w433
              n167 = in-place-cluster #16(w436) -> ("Elapsed Time"=w437:dbl)  [unwired: 1 out]
              n168 = Get Date/Time In Seconds() -> (seconds since 1Jan1904=w439:timestamp)
              n169 = Subtract(x=w439, y=w437) -> (x-y=w438:timestamp)
              n170 = in-place-cluster #16("Car Wash Indicators.Vehicle Out of Position"=TRUE, "Elapsed Time"=w437) -> (w435:T2)
            }
          }
          frame True {
            # "Current Time"
            n171 = Get Date/Time In Seconds() -> (seconds since 1Jan1904=w446:timestamp)
            n172 = Subtract(x=w446, y=w441) -> (x-y=w450:dbl)
            n173 = Greater?(x=w450, y=5.0) -> (0:w448:bool)
            n174 = case shown="False" w448 {
              tunnel: [States."Air Dry" w462] -> w447
              tunnel: w445 -> [w456 w464]
              tunnel: [w456 w461] -> w444
              tunnel: w443 -> [_ w460]
              tunnel: [w455 w458] -> w442
              tunnel: w441 -> [w455 _]
              frame False {
              }
              frame True {
                n175 = Unbundle By Name(w460) -> ("Wash Options"=w459:refnum<vi>)
                n176 = property on="Air Dry" class="Bool (strict)"(error in=w464, "Value"=FALSE) -> (error out=w463:errorcluster)  [unwired: 1 in, 1 out]
                n177 = call "Find next car wash step.vi"("error in (no error)"=w463, "Control Refnum"=w459) -> ("error out"=w461:errorcluster, "Next Car Wash option"=w462:T5)  [unwired: 8 in]
                n178 = Get Date/Time In Seconds() -> (seconds since 1Jan1904=w458:timestamp)
              }
            }
            n179 = Select(t=0.0, s=w448, f=w450) -> (s? t:f=w449:dbl)
            n180 = in-place {
              in-place-border: w449 -> [w467]
              n181 = in-place-cluster #17(w454) -> ()  [unwired: 3 out]
              n182 = in-place-cluster #17("Car Wash Indicators.Vehicle Out of Position"=FALSE, "Car Wash Indicators.Air Dry"=TRUE ("Car Wash Indicators.Under Body Wash"), "Elapsed Time"=w467) -> (w453:T2)
            }
          }
        }
      }
      frame "Stop" {
        # "Aborts the program\n\nEnables the START and WASH OPTIONS control\nShows that the Was is vacant, resets the elapsed time to 0 and puts the car position slider to 0"
        n183 = Unbundle By Name(w471) -> ("Start"=w490:refnum<vi>, "Wash Options"=w489:refnum<vi>, "Wash Entry"=w485:refnum<vi>, "Elapsed Time"=w483:refnum<vi>, "Car Position Slider"=w480:refnum<vi>)
        n184 = Build Array(w490, w489) -> (w488:refnum<vi>[])
        n185 = call "Enable Disable Controls.vi"("error in (no error)"=w470, "Disabled"=T6."Enabled", "Control Refnum"=w488) -> ("Error Out"=w486:errorcluster)  [unwired: 8 in]
        n186 = property class="Bool (strict)"(reference=w485, error in=w486, "Value"=TRUE, "BoolText.Text"="Wash Vacant" ("Boolean Text.Text"), "Colors [4]"=cluster{u32, u32}[] [{1245026, 1965842}]) -> (error out=w482:errorcluster)  [unwired: 1 out]
        n187 = property class="DigNum (strict)"(reference=w483, error in=w482, "Value"=0.0) -> (error out=w479:errorcluster)  [unwired: 1 out]
        n188 = property class="Slide (strict)"(reference=w480, error in=w479, "Value"=u8 0) -> (error out=w477:errorcluster)  [unwired: 1 out]
      }
      frame "Exit" {
        # "When all the wash steps are executed, it reaches this step"
        n189 = Unbundle By Name(w491) -> ("Car Position Slider"=w502:refnum<vi>)
        n190 = Bundle By Name(cluster=w504, "Car Wash Indicators.Vehicle Out of Position"=TRUE) -> (w497:T2)
        n191 = property class="Slide (strict)"(reference=w502, error in=w501) -> (error out=w495:errorcluster, "Value"=w500:u8)  [unwired: 1 out]
        n192 = Equal?(x=w500, y=u8 4) -> (x = y?=w498:bool)
        n193 = case shown="False" w498 {
          tunnel: w497 -> [w505 w512]
          tunnel: [States."Exit" States."Initialize"] -> w496
          tunnel: [w505 w509] -> w493
          tunnel: w495 -> [w506 w508]
          tunnel: [w506 w508] -> w494
          frame False {
          }
          frame True {
            n194 = Bundle By Name(cluster=w512, "Car Wash Indicators"=T1 {"Under Body Wash"=FALSE, "Bug Remover"=FALSE, "Pre-Soak"=FALSE, "High Pressure Wash"=FALSE, "Low Pressure Wax"=FALSE, "Spot Free Rinse"=FALSE, "Tire Shine Foam"=FALSE, "Air Dry"=FALSE, "Vehicle Out of Position"=FALSE}) -> (w509:T2)
          }
        }
      }
    }
    "Output" <- w18
    n195 = call <vilib>:"Simple Error Handler.vi"("error in (no error)"=w15) -> ("error out"=w14:errorcluster)  [unwired: 4 in, 4 out]
  }
